vi "Clear.vi"(8 "error in (no error)":errorcluster, 11 "Process In":refnum<class "Process.lvclass">) -> (0 "error out":errorcluster)   [LabVIEW 2020, in "Process.lvclass"]
doc: "Clears any resorces allocated during initialization."
uses:
  Process.lvclass
  Process.lvclass/Process.ctl
  <vilib>/Utility/error.llb/Clear Errors.vi
  <vilib>/Utility/error.llb/Error Cluster From Error Code.vi
  <vilib>/ErrorRing/Error Ring.xnode
  Base/Base.lvclass
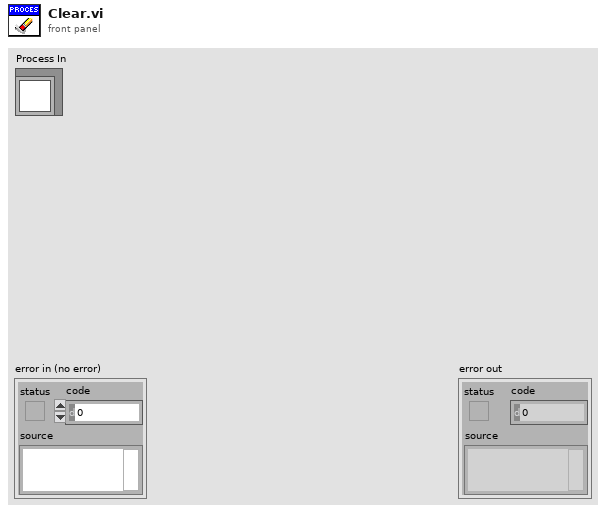
[diagram p1: front panel]
types:
  T1 = typedef "Process.lvclass/Lifecycle State.ctl" = enum16{"Uninitialized", "Initialized", "Started", "Running", "Stopped", "Finished"}
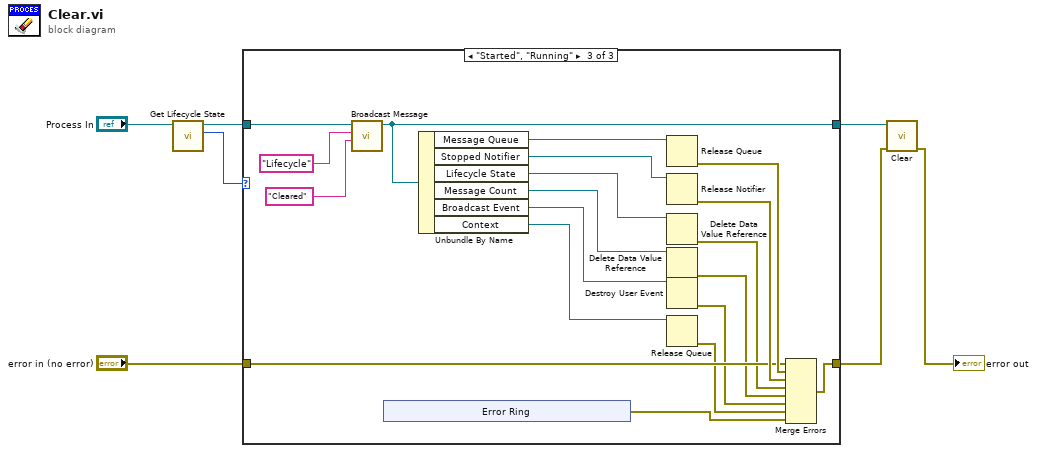
[diagram p0: block diagram]
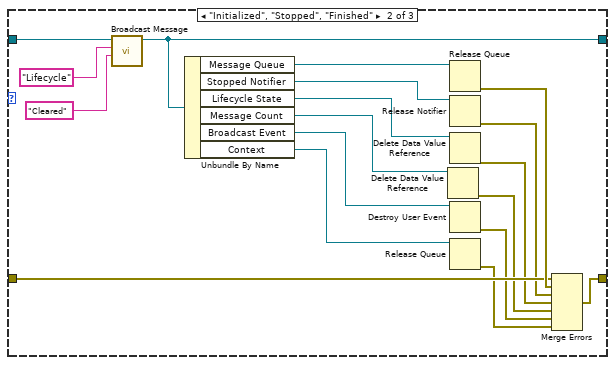
[diagram p3: hidden frame]
diagram:
  n1 = call "Get Lifecycle State.vi"("Process In"="Process In") -> ("Lifecycle State"=w4:T1, "Process Out"=w5:refnum<class "Process.lvclass">)  [unwired: 7 in, 2 out]
  n2 = case shown="\"Started\", \"Running\"" w4 {
    tunnel: [w8 w27 w46] -> w3
    tunnel: [w9 w14 w33] -> w6
    tunnel: w5 -> [w9 w13 w34]
    tunnel: "error in (no error)" -> [w8 w23 w41]
    frame "Uninitialized" {
    }
    frame "Initialized", "Stopped", "Finished" {
      n3 = call-dynamic "Broadcast Message.vi"("Message Data"="Cleared" ("Message"), "Message"="Lifecycle", "Process In"=w13) -> ("Process Out"=w14:refnum<class "Process.lvclass">)  [unwired: 7 in, 1 out]
      n4 = Unbundle By Name(w14) -> ("Message Queue"=w26:refnum<queue>, "Stopped Notifier"=w24:refnum<notifier>, "Lifecycle State"=w22:refnum<data-value>, "Message Count"=w12:refnum<data-value>, "Broadcast Event"=w21:refnum<user-event>, "Context"=w20:refnum<queue>)
      n5 = Delete Data Value Reference(data value reference=w12) -> (error out=w10:errorcluster)  [unwired: 1 in, 1 out]
      n6 = Release Queue(queue=w26) -> (error out=w25:errorcluster)  [unwired: 2 in, 2 out]
      n7 = Release Notifier(notifier=w24) -> (error out=w17:errorcluster)  [unwired: 2 in, 2 out]
      n8 = Delete Data Value Reference(data value reference=w22) -> (error out=w11:errorcluster)  [unwired: 1 in, 1 out]
      n9 = Destroy User Event(user event=w21) -> (error out=w19:errorcluster)  [unwired: 1 in]
      n10 = Release Queue(queue=w20) -> (error out=w18:errorcluster)  [unwired: 2 in, 2 out]
      n11 = Merge Errors(w23, w25, w17, w11, w10, w19, w18) -> (w27:errorcluster)
    }
    frame "Started", "Running" {
      n12 = call-dynamic "Broadcast Message.vi"("Message Data"="Cleared" ("Message"), "Message"="Lifecycle", "Process In"=w34) -> ("Process Out"=w33:refnum<class "Process.lvclass">)  [unwired: 7 in, 1 out]
      n13 = xnode "Error Ring"() -> ("error out"=w35:errorcluster)
      n14 = Unbundle By Name(w33) -> ("Message Queue"=w45:refnum<queue>, "Stopped Notifier"=w43:refnum<notifier>, "Lifecycle State"=w40:refnum<data-value>, "Message Count"=w30:refnum<data-value>, "Broadcast Event"=w38:refnum<user-event>, "Context"=w37:refnum<queue>)
      n15 = Release Queue(queue=w45) -> (error out=w44:errorcluster)  [unwired: 2 in, 2 out]
      n16 = Release Notifier(notifier=w43) -> (error out=w42:errorcluster)  [unwired: 2 in, 2 out]
      n17 = Delete Data Value Reference(data value reference=w40) -> (error out=w29:errorcluster)  [unwired: 1 in, 1 out]
      n18 = Delete Data Value Reference(data value reference=w30) -> (error out=w28:errorcluster)  [unwired: 1 in, 1 out]
      n19 = Destroy User Event(user event=w38) -> (error out=w39:errorcluster)  [unwired: 1 in]
      n20 = Release Queue(queue=w37) -> (error out=w36:errorcluster)  [unwired: 2 in, 2 out]
      n21 = Merge Errors(w41, w44, w42, w29, w28, w39, w36, w35) -> (w46:errorcluster)
    }
  }
  n22 = call-parent "Clear.vi"("error in (no error)"=w3, "Base In"=w6) -> ("error out"=→"error out":errorcluster)  [unwired: 9 in]
